vi "CRYCheck Failed Points.vi"(9 "Low Limit":cluster{dbl, dbl}[](array[cluster]) {"?" format="%.2f"; "?" format="%.2f"}, 10 "Up Limit":cluster{dbl, dbl}[](array[cluster]) {"?" format="%.2f"; "?" format="%.2f"}, 11 "Data":cluster{dbl, dbl}[](array[cluster]) {"?" format="%.2f"; "?" format="%.2f"}) -> (2 "Low Failed_X":dbl[](array[numeric]), 3 "Up Failed_X":dbl[](array[numeric]))   [LabVIEW 2013]
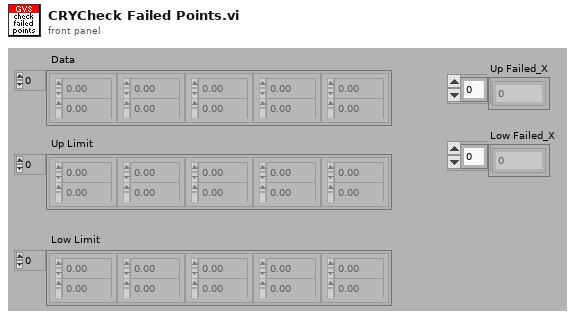
[diagram p1: front panel]
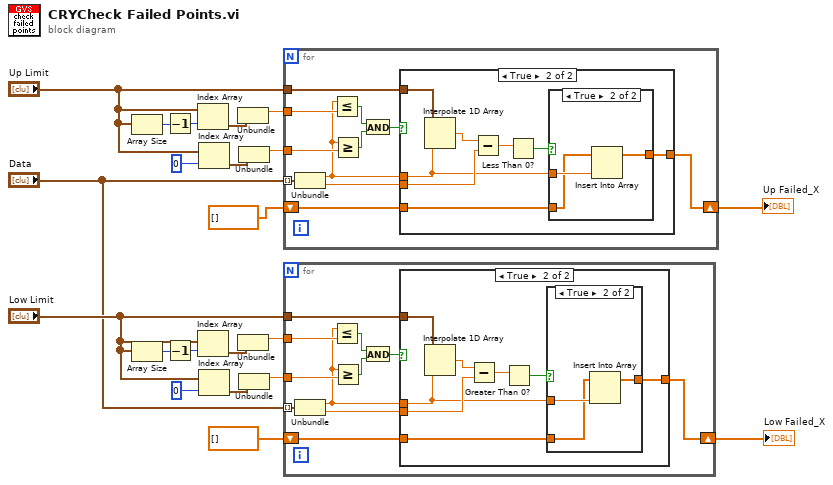
[diagram p0: block diagram]
diagram:
  n1 = Array Size(array="Up Limit") -> (size(s)=w16:i32)
  n2 = Array Size(array="Low Limit") -> (size(s)=w11:i32)
  n3 = Decrement(x=w16) -> (x-1=w17:i32)
  n4 = Decrement(x=w11) -> (x-1=w10:i32)
  n5 = Index Array(array="Up Limit", index=w17) -> (element=w14:cluster{dbl, dbl})
  n6 = Index Array(array="Low Limit", index=w10) -> (element=w13:cluster{dbl, dbl})
  n7 = Index Array(array="Up Limit", index=0) -> (element=w15:cluster{dbl, dbl})
  n8 = Index Array(array="Low Limit", index=0) -> (element=w12:cluster{dbl, dbl})
  n9 = Unbundle(w14) -> (w20:dbl)  [unwired: 1 out]
  n10 = Unbundle(w13) -> (w7:dbl)  [unwired: 1 out]
  n11 = Unbundle(w15) -> (w19:dbl)  [unwired: 1 out]
  n12 = Unbundle(w12) -> (w8:dbl)  [unwired: 1 out]
  n13 = for {
    tunnel: w19 -> [w29]
    tunnel: "Data" -> [w32] mode=indexing
    tunnel: "Up Limit" -> [w31]
    tunnel: w20 -> [w28]
    shift-right: [w22] -> w3
    shift-left: dbl[] [] ("Up Failed") -> [w23]
    n14 = Unbundle(w32) -> (w24:dbl, w30:dbl)
    n15 = Less Or Equal?(x=w24, y=w28) -> (x <= y?=w27:bool)
    n16 = Greater Or Equal?(x=w24, y=w29) -> (x >= y?=w26:bool)
    n17 = And(x=w27, y=w26) -> (x .and. y?=w25:bool)
    n18 = case shown="True" w25 {
      tunnel: w31 -> [_ w41]
      tunnel: w24 -> [_ w36]
      tunnel: w30 -> [_ w39]
      tunnel: w23 -> [w33 w35]
      tunnel: [w33 w34] -> w22
      frame False {
      }
      frame True {
        n19 = Interpolate 1D Array(1:w36, 2:w41) -> (0:w40:dbl)
        n20 = Subtract(x=w40, y=w39) -> (x-y=w38:dbl)
        n21 = Less Than 0?(x=w38) -> (x < 0?=w37:bool)
        n22 = case shown="True" w37 {
          tunnel: w36 -> [_ w45]
          tunnel: w35 -> [w42 w44]
          tunnel: [w42 w43] -> w34
          frame False {
          }
          frame True {
            n23 = Insert Into Array(array=w44, new element=w45) -> (w43:dbl[])  [unwired: 1 in]
          }
        }
      }
    }
  }
  "Up Failed_X" <- w3
  n24 = for {
    tunnel: w8 -> [w53]
    tunnel: "Data" -> [w56] mode=indexing
    tunnel: "Low Limit" -> [w55]
    tunnel: w7 -> [w52]
    shift-right: [w46] -> w1
    shift-left: dbl[] [] ("Up Failed") -> [w47]
    n25 = Unbundle(w56) -> (w48:dbl, w54:dbl)
    n26 = Less Or Equal?(x=w48, y=w52) -> (x <= y?=w51:bool)
    n27 = Greater Or Equal?(x=w48, y=w53) -> (x >= y?=w50:bool)
    n28 = And(x=w51, y=w50) -> (x .and. y?=w49:bool)
    n29 = case shown="True" w49 {
      tunnel: w55 -> [_ w65]
      tunnel: w48 -> [_ w60]
      tunnel: w54 -> [_ w63]
      tunnel: w47 -> [w57 w59]
      tunnel: [w57 w58] -> w46
      frame False {
      }
      frame True {
        n30 = Interpolate 1D Array(1:w60, 2:w65) -> (0:w64:dbl)
        n31 = Subtract(x=w64, y=w63) -> (x-y=w62:dbl)
        n32 = Greater Than 0?(x=w62) -> (x > 0?=w61:bool)
        n33 = case shown="True" w61 {
          tunnel: w60 -> [_ w69]
          tunnel: w59 -> [w66 w68]
          tunnel: [w66 w67] -> w58
          frame False {
          }
          frame True {
            n34 = Insert Into Array(array=w68, new element=w69) -> (w67:dbl[])  [unwired: 1 in]
          }
        }
      }
    }
  }
  "Low Failed_X" <- w1
